vi "Start.vi"(8 "error in (no error)":errorcluster, 11 "FGen PXI Base CFG in":refnum<class "FGen PXI Base CFG.lvclass">) -> (0 "error out":errorcluster, 3 "FGen PXI Base CFG out":refnum<class "FGen PXI Base CFG.lvclass">)   [LabVIEW 2023, in "FGen PXI Base CFG.lvlib" / "FGen PXI Base CFG.lvclass"]
uses:
  FGen PXI Base CFG.lvclass
  FGen PXI Base CFG.lvclass/FGen PXI Base CFG.ctl
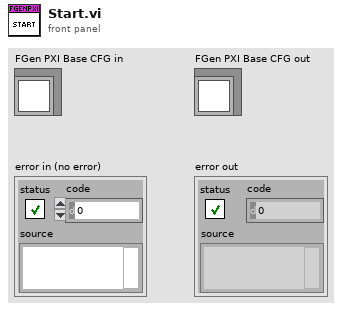
[diagram p1: front panel]
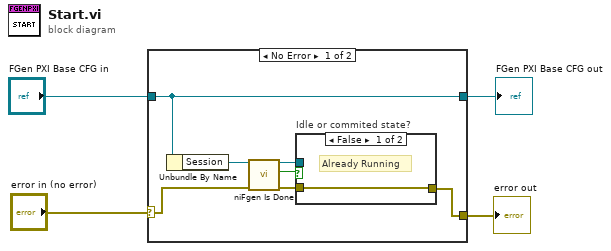
[diagram p0: block diagram]
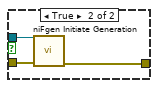
[diagram p2: hidden frame]
diagram:
  n1 = case shown="No Error" "error in (no error)" {
    selector: "error in (no error)" -> [w8 w16]
    tunnel: "FGen PXI Base CFG in" -> [w9 w15]
    tunnel: [w10 w16] -> w3
    tunnel: [w9 w15] -> w1
    frame No Error {
      n2 = Unbundle By Name(w9) -> ("Session"=w7:refnum<k15>)
      n3 = call <instrlib>:"niFgen Is Done.vi"("error in (no error)"=w8, "Instrument Handle"=w7) -> ("error out"=w5:errorcluster, "Done"=w6:bool)  [unwired: 7 in, 1 out]
      n4 = case "Idle or commited state?" shown="False" w6 {
        tunnel: [w11 w14] -> w10
        tunnel: w7 -> [_ w13]
        tunnel: w5 -> [w11 w12]
        frame False {
          # "Already Running"
        }
        frame True {
          n5 = call <instrlib>:"niFgen Initiate Generation.vi"("error in (no error)"=w12, "Instrument Handle"=w13) -> ("error out"=w14:errorcluster)  [unwired: 8 in, 1 out]
        }
      }
    }
    frame Error {
    }
  }
  "error out" <- w3
  "FGen PXI Base CFG out" <- w1
